vi "Anritsu VNA Set Channel.vi"(7 "Anritsu VNA":T1, 8 "error in (no error)":errorcluster, 10 "Channel":i8=1 min=1 step=1, 11 "VISA Resource Name":refnum<visa-resource-name>) -> (0 "error out":errorcluster, 3 "dup VISA Resource Name":refnum<visa-resource-name>)   [LabVIEW 2011]
uses:
  TypeDefs/Anritsu VNA Instrument Info.ctl
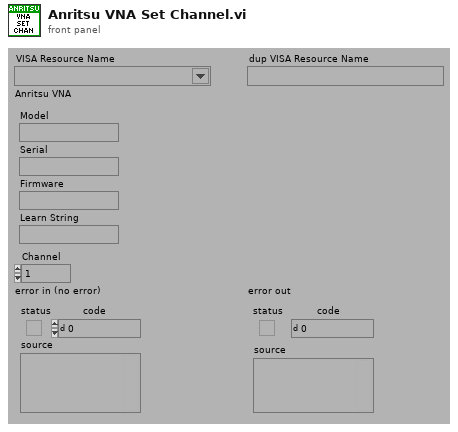
[diagram p1: front panel]
types:
  T1 = typedef "Anritsu VNA Instrument Info.ctl" = cluster{"Model":string, "Serial":string, "Firmware":string, "Learn String":string}
  T2 = typedef "Anritsu VNA Model.ctl" = enum16{"Not Supported", "37XXXX", "MS20XXX", "MS462XX", "MS464XX"}
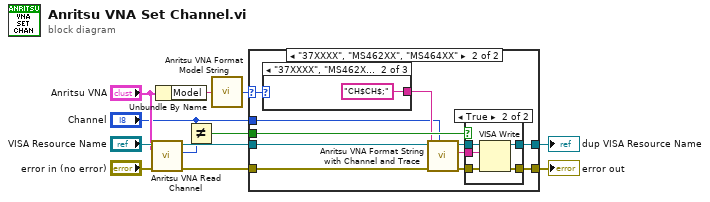
[diagram p0: block diagram]
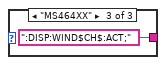
[diagram p5: hidden frame]
diagram:
  n1 = call "Anritsu VNA Read Channel.vi"("Anritsu VNA"="Anritsu VNA", "error in (no error)"="error in (no error)", "VISA Resource Name"="VISA Resource Name") -> ("error out"=w8:errorcluster, "Channel"=w5:i8, "dup VISA Resource Name"=w7:refnum<visa-resource-name>)  [unwired: 6 out]
  n2 = Unbundle By Name("Anritsu VNA") -> ("Model"=w3:string)
  n3 = Not Equal?(x="Channel", y=w5) -> (x != y?=w1:bool)
  n4 = call "Anritsu VNA Format Model String.vi"("Model"=w3) -> ("Model"=w2:T2)
  n5 = case shown="\"37XXXX\", \"MS462XX\", \"MS464XX\"" w2 {
    selector: w2 -> [_ w23]
    tunnel: [w13 w20] -> w12
    tunnel: [w14 w19] -> w11
    tunnel: "Channel" -> [_ w15]
    tunnel: w7 -> [w13 w22]
    tunnel: w8 -> [w14 w21]
    tunnel: w1 -> [_ w18]
    frame "Not Supported", "MS20XXX" {
      # "These VNAs don't have multiple channels."
    }
    frame "37XXXX", "MS462XX", "MS464XX" {
      n6 = case shown="\"37XXXX\", \"MS462XX\"" w23 {
        tunnel: [_ "CH$CH$;" ":DISP:WIND$CH$:ACT;"] -> w16
        frame "Not Supported", "MS20XXX" {
        }
        frame "37XXXX", "MS462XX" {
        }
        frame "MS464XX" {
        }
      }
      n7 = call "Anritsu VNA Format String with Channel and Trace.vi"("Channel"=w15, "String"=w16) -> ("String Out"=w17:string)  [unwired: 1 in, 6 out]
      n8 = case shown="True" w18 {
        tunnel: w22 -> [w25 w30]
        tunnel: w21 -> [w24 w29]
        tunnel: [w25 w28] -> w20
        tunnel: [w24 w27] -> w19
        tunnel: w17 -> [_ w26]
        frame False {
        }
        frame True {
          n9 = VISA Write(VISA resource name=w30, write buffer=w26, error in (no error)=w29) -> (VISA resource name out=w28:refnum<visa-resource-name>, error out=w27:errorcluster)  [unwired: 1 out]
        }
      }
    }
  }
  "dup VISA Resource Name" <- w12
  "error out" <- w11
